vi "IPv4-Parse.vi"(11 "IPv4 Packet (in)":u8[](array[numeric])=[69, 0, 0, 60, 12, 166, 0, 0, 128, 1, 169, 57, 192, 168, 1, 200, 192, 168, 1, 201, 8, 0, 77, 77, 0, 1, 0, 14, 97, 98, 99, 100, 101, 102, 103, 104, 105, 106, 107, 108, 109, 110, 111, 112, 113, 114, 115, 116, 117, 118, 119, 97, 98, 99, 100, 101, 102, 103, 104, 105] format="%02x") -> (1 "Header\nChecksum\nOk?":bool=TRUE, 2 "IPv4 Payload":u8[](array[numeric])=[8, 0, 77, 77, 0, 1, 0, 14, 97, 98, 99, 100, 101, 102, 103, 104, 105, 106, 107, 108, 109, 110, 111, 112, 113, 114, 115, 116, 117, 118, 119, 97, 98, 99, 100, 101, 102, 103, 104, 105] format="%02x", 3 "Header":T1)   [LabVIEW 2017]
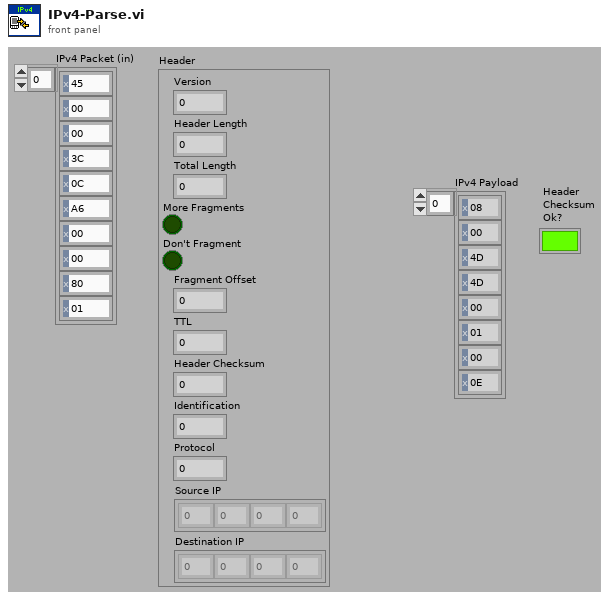
[diagram p1: front panel]
types:
  T1 = cluster{"Version":u8, "Header Length":u8, "Total Length":u16, "More Fragments":bool, "Don't Fragment":bool, "Fragment Offset":u16, "TTL":u8, "Header Checksum":u16, "Identification":u16, "Protocol":u8, "Source IP":u8[], "Destination IP":u8[]}
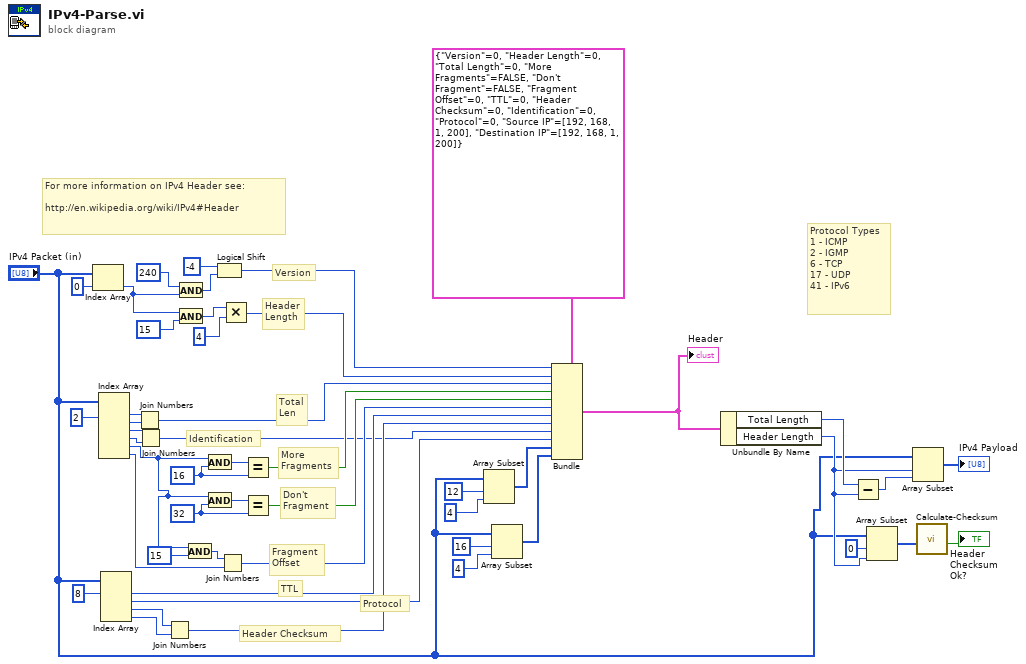
[diagram p0: block diagram]
diagram:
  w42 = u8 32 ("y")
  w40 = u8 16 ("y")
  # "Protocol Types\n1 - ICMP\n2 - IGMP\n6 - TCP\n17 - UDP\n41 - IPv6"
  # "Identification"
  # "Header Checksum"
  # "Protocol"
  # "TTL"
  # "Don't\nFragment"
  # "More\nFragments"
  # "Fragment\nOffset"
  # "Total\nLen"
  # "Header\nLength"
  # "Version"
  # "For more information on IPv4 Header see:\n\nhttp://en.wikipedia.org/wiki/IPv4#Header"
  n1 = Index Array(array="IPv4 Packet (in)", index=0) -> (element=w10:u8)
  n2 = Index Array(array="IPv4 Packet (in)", index #1=2 ("index")) -> (element #1=w24:u8, element #2=w23:u8, element #3=w25:u8, element #4=w26:u8, element #5=w44:u8, element #6=w27:u8)  [unwired: 5 in]
  n3 = Index Array(array="IPv4 Packet (in)", index #1=8 ("index")) -> (element #1=w47:u8, element #2=w16:u8, element #3=w31:u8, element #4=w32:u8)  [unwired: 3 in]
  n4 = Join Numbers(hi=w24, lo=w23) -> ((hi.lo)=w7:u16)
  n5 = Join Numbers(hi=w25, lo=w26) -> ((hi.lo)=w9:u16)
  n6 = Join Numbers(hi=w31, lo=w32) -> ((hi.lo)=w48:u16)
  n7 = And(x=u8 240 ("y"), y=w10) -> (x .and. y?=w13:u8)
  n8 = And(x=w10, y=u8 15) -> (x .and. y?=w20:u8)
  n9 = And(x=w44, y=u8 15) -> (x .and. y?=w29:u8)
  n10 = And(x=w44, y=w40) -> (x .and. y?=w39:u8)
  n11 = And(x=w44, y=w42) -> (x .and. y?=w43:u8)
  n12 = Logical Shift(y=i8 -4, x=w13) -> (x << y=w12:u8)
  n13 = Join Numbers(hi=w29, lo=w27) -> ((hi.lo)=w46:u16)
  n14 = Multiply(x=w20, y=u8 4) -> (x*y=w6:u8)
  n15 = Equal?(x=w39, y=w40) -> (x = y?=w41:bool)
  n16 = Equal?(x=w43, y=w42) -> (x = y?=w45:bool)
  n17 = Array Subset(array="IPv4 Packet (in)", index=12, length=4) -> (w3:u8[])
  n18 = Array Subset(array="IPv4 Packet (in)", index=16, length=4) -> (w2:u8[])
  n19 = Bundle(cluster=T1 {"Version"=0, "Header Length"=0, "Total Length"=0, "More Fragments"=FALSE, "Don't Fragment"=FALSE, "Fragment Offset"=0, "TTL"=0, "Header Checksum"=0, "Identification"=0, "Protocol"=0, "Source IP"=[192, 168, 1, 200], "Destination IP"=[192, 168, 1, 200]} ("Header"), "Version"=w12, "Header Length"=w6, "Total Length"=w7, "More Fragments"=w41, "Don't Fragment"=w45, "Fragment Offset"=w46, "TTL"=w47, "Header Checksum"=w48, "Identification"=w9, "Protocol"=w16, "Source IP"=w3, "Destination IP"=w2) -> (w8:T1)
  "Header" <- w8
  n20 = Unbundle By Name(w8) -> ("Total Length"=w5:u16, "Header Length"=w4:u8)
  n21 = Subtract(x=w5, y=w4) -> (x-y=w38:u16)
  n22 = Array Subset(array="IPv4 Packet (in)", index=0, length=w4) -> (w50:u8[])
  n23 = Array Subset(array="IPv4 Packet (in)", index=w4, length=w38) -> (→"IPv4 Payload":u8[])
  n24 = call "Calculate-Checksum.vi"("Array"=w50) -> ("Checksum OK?"=→"Header\nChecksum\nOk?":bool)  [unwired: 9 in, 1 out]
